vi "Parse Data.vi"(8 "error in (no error)":errorcluster, 10 "R/W?":T1, 11 "Data in":string) -> (0 "error out":errorcluster, 3 "Data out":u16)   [LabVIEW 2018, in "Config_Read_SPI.lvclass"]
uses:
  Config_Read_SPI.lvclass
  Classes/Config_Read/RW_Option.ctl
  Classes/Config_Read/Config_Read_BML.lvclass
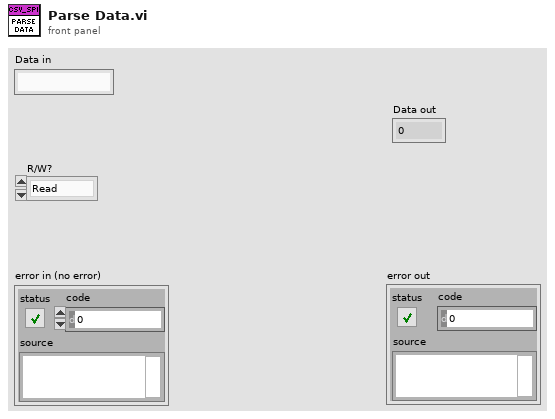
[diagram p1: front panel]
types:
  T1 = typedef "Config_Read_BML.lvclass/RW_Option.ctl" = enum16{"Read", "Write", "R/W"}
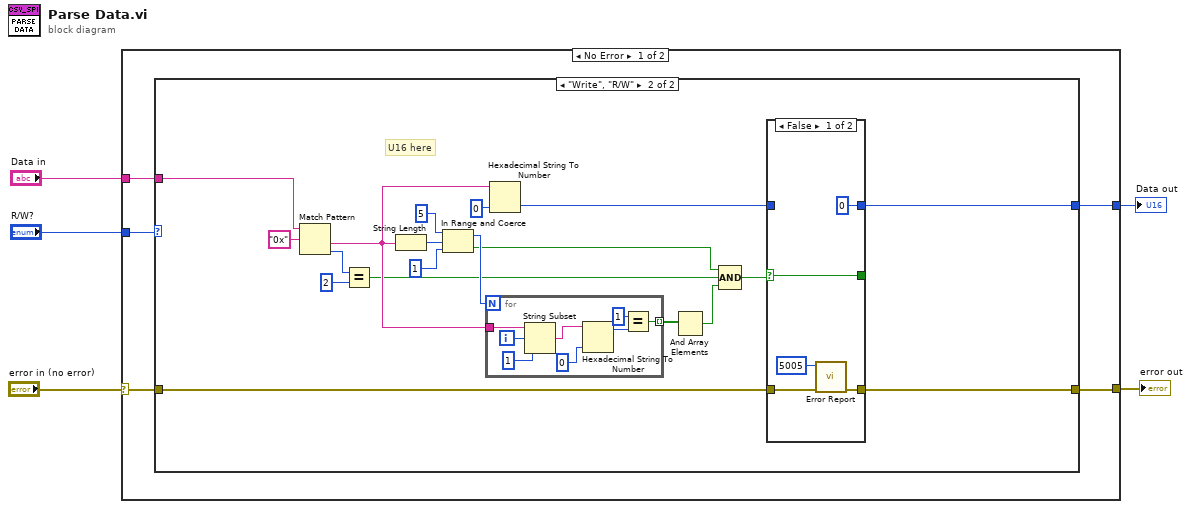
[diagram p0: block diagram]
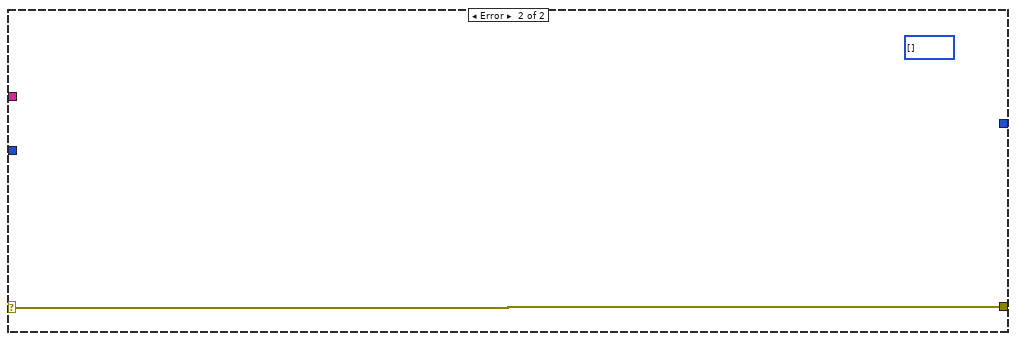
[diagram p4: hidden frame]
diagram:
  n1 = case shown="No Error" "error in (no error)" {
    selector: "error in (no error)" -> [w9 w47]
    tunnel: "Data in" -> [w10 _]
    tunnel: [w8 w47] -> w3
    tunnel: "R/W?" -> [w7 _]
    tunnel: [w6 _] -> w1
    frame No Error {
      n2 = case shown="\"Write\", \"R/W\"" w7 {
        tunnel: w10 -> [_ w30]
        tunnel: w9 -> [w11 w29]
        tunnel: [w11 w13] -> w8
        tunnel: [_ w12] -> w6
        frame "Read", Default {
        }
        frame "Write", "R/W" {
          # "U16 here"
          n3 = Match Pattern(string=w30, regular expression="0x") -> (after substring=w26:string, offset past match=w17:i32)  [unwired: 1 in, 2 out]
          n4 = Equal?(x=w17, y=2) -> (x = y?=w20:bool)
          n5 = String Length(string=w26) -> (length=w21:i32)
          n6 = In Range and Coerce(upper limit=5, x=w21, lower limit=1 ("upper limit")) -> (coerced(x)=w25:i32, In Range?=w24:bool)
          n7 = for {
            N: w25 -> [_]
            tunnel: w26 -> [w46]
            tunnel: [w39] -> w27 mode=indexing
            i -> [w45]
            n8 = String Subset(string=w46, offset (0)=w45, length (rest)=1 ("length (rest)")) -> (substring=w43:string)
            n9 = Hexadecimal String To Number(string=w43, default (0uL)=u8 0 ("Addr out")) -> (offset past number=w41:i32)  [unwired: 1 in, 1 out]
            n10 = Equal?(x=1, y=w41) -> (x = y?=w39:bool)
          }
          n11 = Hexadecimal String To Number(string=w26, default (0uL)=u16 0 ("Addr out")) -> (number=w14:u16)  [unwired: 1 in, 1 out]
          n12 = And Array Elements(Boolean array=w27) -> (logical AND=w28:bool)
          n13 = Compound Arithmetic op=AND(w24, w20, w28) -> (w15:bool)
          n14 = case shown="False" w15 {
            selector: w15 -> [w33 w37]
            tunnel: w14 -> [_ w36]
            tunnel: w29 -> [w32 w38]
            tunnel: [w34 w38] -> w13
            tunnel: [w33 w37] -> _
            tunnel: [u16 0 w36] -> w12
            frame False {
              n15 = call "Error Report.vi"("error in (no error)"=w32, "Error Code"=i16 5005) -> ("error out"=w34:errorcluster)  [unwired: 9 in]
            }
            frame True {
            }
          }
        }
      }
    }
    frame Error {
      (unwired) u8[] []
    }
  }
  "error out" <- w3
  "Data out" <- w1
